vi "ST5 Home Search.vi"(0 "Port COM":refnum<visa-resource-name>, 5 "Home Dir":bool, 7 "Home Speed Par":T1={"Vitesse (Tour/s)"=0.5, "Accél"=2.0, "Décél"=2.0} {"Décél" min=0.01 max=20.0 step=0.01 format="%#.3g"; "Accél" min=0.01 max=20.0 step=0.01 format="%#.3g"; "Vitesse (Tour/s)" min=0.01 max=20.0 step=0.01 format="%#.4g"}, 9 "Ext Stop Ref":refnum<vi>, 11 "error in (no error)":errorcluster, 12 "HomeInput":u8=1 caption="Home Input" min=1 max=8 step=1, 13 "Normal Speed Par":T1={"Vitesse (Tour/s)"=1.0, "Accél"=2.0, "Décél"=2.0} {"Décél" min=0.01 max=20.0 step=0.01 format="%#.3g"; "Accél" min=0.01 max=20.0 step=0.01 format="%#.3g"; "Vitesse (Tour/s)" min=0.01 max=20.0 step=0.01 format="%#.4g"}) -> (4 "Port COM Out":refnum<visa-resource-name>, 6 "CW Limit":bool, 8 "CCW Limit":bool, 10 "Alarme":u32, 15 "error out":errorcluster)   [LabVIEW 2019]
doc: "Ce Vi envoie les chaînes de commande au contrôlleur de moteur ST5-Q et vérifie si une réponse se trouve dans le buffer du port série"
uses:
  <userlib>/ST5/HomeViStates.ctl
panel:
  in  "Stop":bool
  out "Status":T2
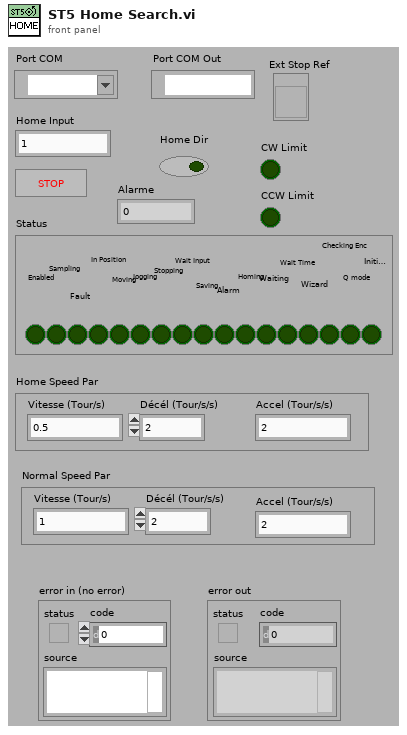
[diagram p1: front panel]
types:
  T1 = cluster{"Vitesse (Tour/s)":dbl, "Accél":dbl, "Décél":dbl}
  T2 = cluster{"Enabled":bool, "Sampling":bool, "Fault":bool, "In Position":bool, "Moving":bool, "Jogging":bool, "Stopping":bool, "Wait Input":bool, "Saving":bool, "Alarm":bool, "Homing":bool, "Waiting":bool, "Wait Time":bool, "Wizard":bool, "Checking Enc":bool, "Q mode":bool, "Initializing":bool}
  T3 = typedef "HomeViStates.ctl" = enum16{"SetHomeSpeed", "Read", "ReturnNormPar", "End"}
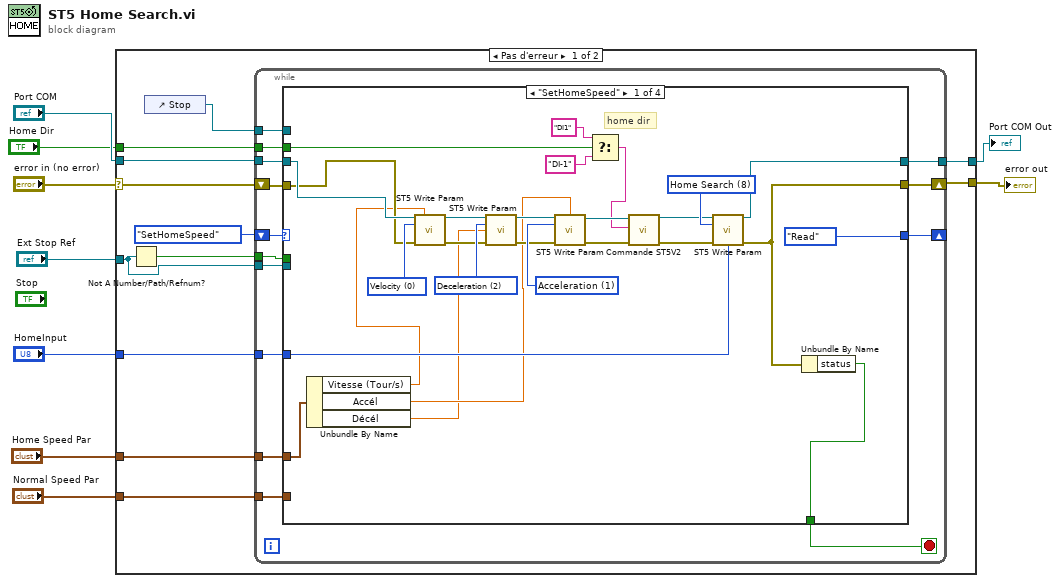
[diagram p0: block diagram]
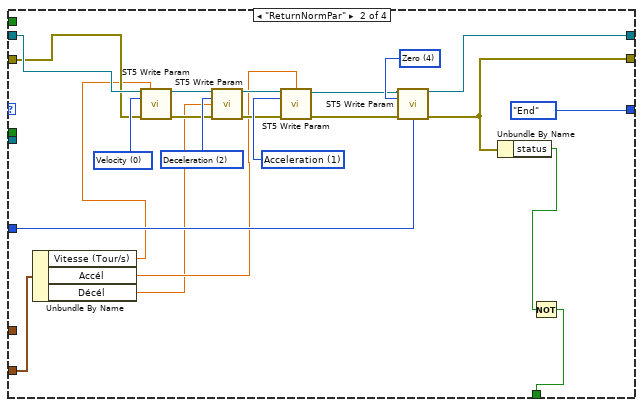
[diagram p2: hidden frame]
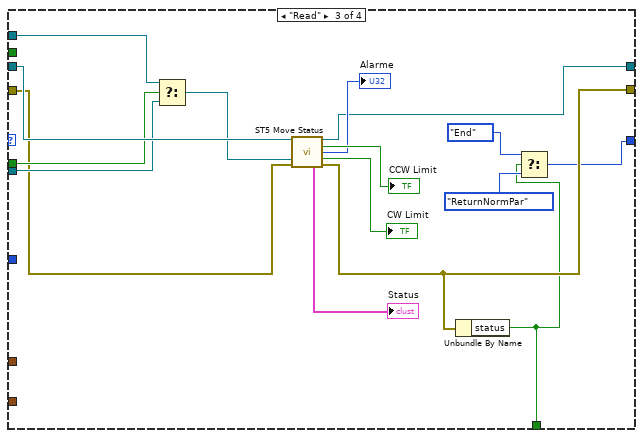
[diagram p3: hidden frame]
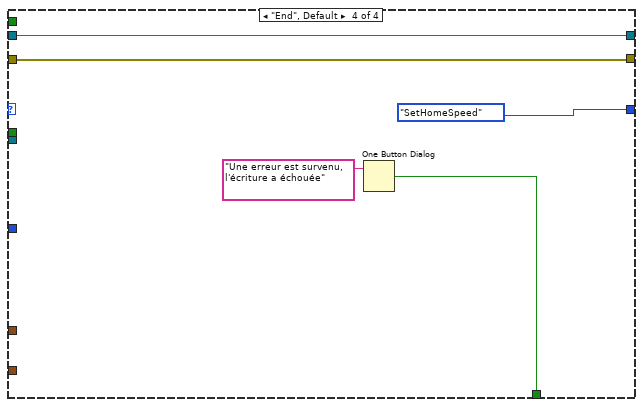
[diagram p4: hidden frame]
diagram:
  n1 = case shown="Pas d'erreur" "error in (no error)" {
    selector: "error in (no error)" -> [w20 w107]
    tunnel: "Port COM" -> [w21 w106]
    tunnel: [w18 w107] -> w1
    tunnel: [w17 w106] -> w7
    tunnel: "HomeInput" -> [w16 _]
    tunnel: "Ext Stop Ref" -> [w15 _]
    tunnel: "Home Speed Par" -> [w12 _]
    tunnel: "Home Dir" -> [w11 _]
    tunnel: "Normal Speed Par" -> [w10 _]
    frame No Error {
      n2 = Not A Number/Path/Refnum?(number/path/refnum=w15) -> (NaN/Path/Refnum?=w14:bool)
      n3 = control-ref of="Stop"() -> (w13:refnum<vi>)
      n4 = while {
        tunnel: w21 -> [w35]
        shift-right: [w32] -> w18
        shift-left: w20 -> [w34]
        shift-right: [w31] -> _
        shift-left: HomeViStates."SetHomeSpeed" ("Énum") -> [w33]
        tunnel: [w29] -> w17
        tunnel: w16 -> [w28]
        tunnel: w15 -> [w27]
        tunnel: w14 -> [w26]
        tunnel: w13 -> [w25]
        tunnel: w12 -> [w24]
        tunnel: w11 -> [w23]
        tunnel: w10 -> [w22]
        stop <- w30 stop-if-true
        n5 = case shown="\"SetHomeSpeed\"" w33 {
          tunnel: w35 -> [w54 w77 w96 w102]
          tunnel: w34 -> [w48 w71 w91 w105]
          tunnel: [w50 w73 w89 w105] -> w32
          tunnel: [HomeViStates."Read" ("Énum") HomeViStates."End" ("Énum") w86 HomeViStates."SetHomeSpeed" ("Énum")] -> w31
          tunnel: [w62 w64 w85 w103] -> w30
          tunnel: [w49 w72 w92 w102] -> w29
          tunnel: w28 -> [w51 w74 _ _]
          tunnel: w27 -> [_ _ w93 _]
          tunnel: w26 -> [_ _ w95 _]
          tunnel: w25 -> [_ _ w94 _]
          tunnel: w24 -> [w47 _ _ _]
          tunnel: w23 -> [w38 _ _ _]
          tunnel: w22 -> [_ w68 _ _]
          frame "SetHomeSpeed" {
            w52 = u16 8 items=["Velocity", "Acceleration", "Deceleration", "Max Acceleration", "Zero", "Save", "Encoder Res", "Clear Alarm", "Home Search", "Motor Enable", "Motor Disable"] ("Parameters")
            w57 = u16 1 items=["Velocity", "Acceleration", "Deceleration", "Max Acceleration", "Zero", "Save", "Encoder Res", "Clear Alarm", "Home Search", "Motor Enable", "Motor Disable"] ("Parameters")
            w58 = u16 2 items=["Velocity", "Acceleration", "Deceleration", "Max Acceleration", "Zero", "Save", "Encoder Res", "Clear Alarm", "Home Search", "Motor Enable", "Motor Disable"] ("Parameters")
            w59 = u16 0 items=["Velocity", "Acceleration", "Deceleration", "Max Acceleration", "Zero", "Save", "Encoder Res", "Clear Alarm", "Home Search", "Motor Enable", "Motor Disable"] ("Parameters")
            # "home dir"
            n6 = Unbundle By Name(w47) -> ("Vitesse (Tour/s)"=w36:dbl, "Accél"=w46:dbl, "Décél"=w45:dbl)
            n7 = call <userlib>:"ST5 Write Param.vi"("Port COM"=w54, "Vitesse"=w36, "Parameters"=w59, "error in (no error)"=w48) -> ("Port COM Out"=w61:refnum<visa-resource-name>, "error out"=w56:errorcluster)  [unwired: 10 in]
            n8 = call <userlib>:"ST5 Write Param.vi"("Port COM"=w61, "Parameters"=w58, "Décél"=w45, "error in (no error)"=w56) -> ("Port COM Out"=w60:refnum<visa-resource-name>, "error out"=w55:errorcluster)  [unwired: 10 in]
            n9 = call <userlib>:"ST5 Write Param.vi"("Port COM"=w60, "Accél"=w46, "Parameters"=w57, "error in (no error)"=w55) -> ("Port COM Out"=w41:refnum<visa-resource-name>, "error out"=w44:errorcluster)  [unwired: 10 in]
            n10 = Select(t="DI1" ("Commande"), s=w38, f="DI-1" ("Commande")) -> (s? t:f=w37:string)
            n11 = call <userlib>:"Commande ST5V2.vi"("error in (no error)"=w44, "Commande"=w37, "Port COM"=w41) -> ("error out"=w43:errorcluster, "Port Out"=w42:refnum<visa-resource-name>)  [unwired: 1 in, 2 out]
            n12 = call <userlib>:"ST5 Write Param.vi"("Port COM"=w42, "Parameters"=w52, "error in (no error)"=w43, "HomeInput"=w51) -> ("Port COM Out"=w49:refnum<visa-resource-name>, "error out"=w50:errorcluster)  [unwired: 10 in]
            n13 = Unbundle By Name(w50) -> ("status"=w62:bool)
          }
          frame "ReturnNormPar" {
            w75 = u16 4 items=["Velocity", "Acceleration", "Deceleration", "Max Acceleration", "Zero", "Save", "Encoder Res", "Clear Alarm", "Home Search", "Motor Enable", "Motor Disable"] ("Parameters")
            w80 = u16 1 items=["Velocity", "Acceleration", "Deceleration", "Max Acceleration", "Zero", "Save", "Encoder Res", "Clear Alarm", "Home Search", "Motor Enable", "Motor Disable"] ("Parameters")
            w81 = u16 2 items=["Velocity", "Acceleration", "Deceleration", "Max Acceleration", "Zero", "Save", "Encoder Res", "Clear Alarm", "Home Search", "Motor Enable", "Motor Disable"] ("Parameters")
            w82 = u16 0 items=["Velocity", "Acceleration", "Deceleration", "Max Acceleration", "Zero", "Save", "Encoder Res", "Clear Alarm", "Home Search", "Motor Enable", "Motor Disable"] ("Parameters")
            n14 = Unbundle By Name(w68) -> ("Vitesse (Tour/s)"=w63:dbl, "Accél"=w70:dbl, "Décél"=w69:dbl)
            n15 = call <userlib>:"ST5 Write Param.vi"("Port COM"=w77, "Vitesse"=w63, "Parameters"=w82, "error in (no error)"=w71) -> ("Port COM Out"=w84:refnum<visa-resource-name>, "error out"=w79:errorcluster)  [unwired: 10 in]
            n16 = call <userlib>:"ST5 Write Param.vi"("Port COM"=w84, "Parameters"=w81, "Décél"=w69, "error in (no error)"=w79) -> ("Port COM Out"=w83:refnum<visa-resource-name>, "error out"=w78:errorcluster)  [unwired: 10 in]
            n17 = call <userlib>:"ST5 Write Param.vi"("Port COM"=w83, "Accél"=w70, "Parameters"=w80, "error in (no error)"=w78) -> ("Port COM Out"=w66:refnum<visa-resource-name>, "error out"=w67:errorcluster)  [unwired: 10 in]
            n18 = call <userlib>:"ST5 Write Param.vi"("Port COM"=w66, "Parameters"=w75, "error in (no error)"=w67, "HomeInput"=w74) -> ("Port COM Out"=w72:refnum<visa-resource-name>, "error out"=w73:errorcluster)  [unwired: 10 in]
            n19 = Unbundle By Name(w73) -> ("status"=w65:bool)
            n20 = Not(x=w65) -> (.not. x?=w64:bool)
          }
          frame "Read" {
            n21 = Select(t=w94, s=w95, f=w93) -> (s? t:f=w90:refnum<vi>)
            n22 = call <userlib>:"ST5 Move Status.vi"("Port COM"=w96, "Stop Ref"=w90, "error in"=w91) -> ("Port Out"=w92:refnum<visa-resource-name>, "CCW Limit"=→"CCW Limit":bool, "Alarme"=→"Alarme":u32, "CW Limit"=→"CW Limit":bool, "Status"=→"Status":T2, "error out"=w89:errorcluster)  [unwired: 7 in]
            n23 = Unbundle By Name(w89) -> ("status"=w85:bool)
            n24 = Select(t=HomeViStates."End" ("Énum"), s=w85, f=HomeViStates."ReturnNormPar" ("Énum")) -> (s? t:f=w86:T3)
          }
          frame "End", Default {
            n25 = One Button Dialog(message="Une erreur est survenu, l'écriture a échouée") -> (true=w103:bool)  [unwired: 1 in]
          }
        }
      }
    }
    frame Error {
    }
  }
  "Port COM Out" <- w7
  "error out" <- w1
